vi "Estiban Shooter Code.vi"(9 "Cannon Height in Inches":dbl, 10 "Target Height in Inches":dbl, 11 "Distance to Shoot In Feet":dbl) -> (3 "Wheel RPM":dbl)   [LabVIEW 2011]
panel:
  out "Wheel RPS":dbl
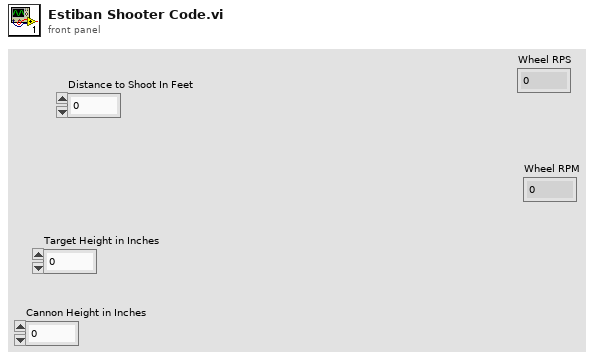
[diagram p1: front panel]
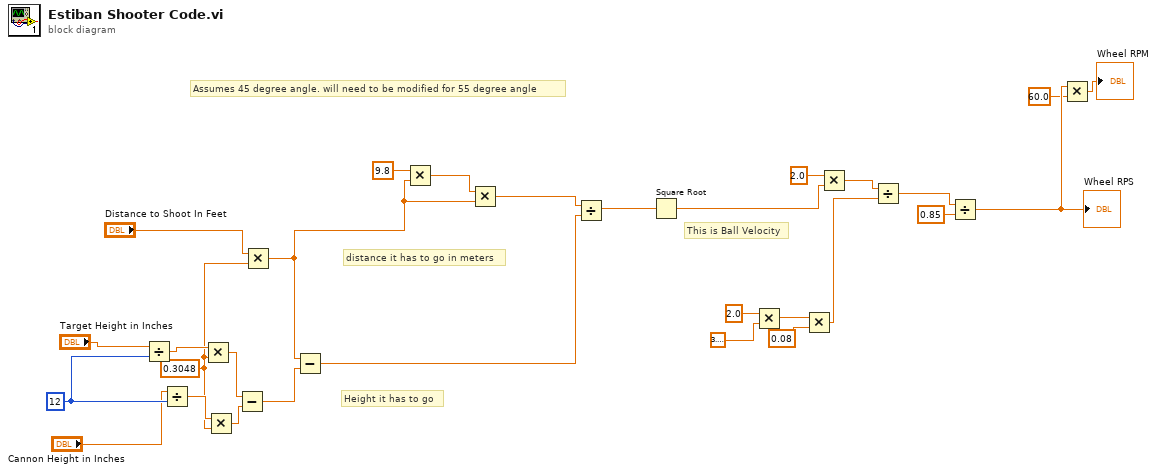
[diagram p0: block diagram]
diagram:
  w14 = 0.3048 ("y")
  w27 = 12
  # "distance it has to go in meters"
  # "Height it has to go"
  # "Assumes 45 degree angle. will need to be modified for 55 degree angle"
  # "This is Ball Velocity"
  n1 = Divide(x="Target Height in Inches", y=w27) -> (x/y=w25:dbl)
  n2 = Divide(x="Cannon Height in Inches", y=w27) -> (x/y=w22:dbl)
  n3 = Multiply(x=w25, y=w14) -> (x*y=w24:dbl)
  n4 = Multiply(x=w22, y=w14) -> (x*y=w23:dbl)
  n5 = Subtract(x=w24, y=w23) -> (x-y=w29:dbl)
  n6 = Multiply(x="Distance to Shoot In Feet", y=w14) -> (x*y=w15:dbl)
  n7 = Subtract(x=w15, y=w29) -> (x-y=w18:dbl)
  n8 = Multiply(x=9.8, y=w15) -> (x*y=w20:dbl)
  n9 = Multiply(x=w20, y=w15) -> (x*y=w19:dbl)
  n10 = Divide(x=w19, y=w18) -> (x/y=w17:dbl)
  n11 = Square Root(x=w17) -> (sqrt(x)=w12:dbl)
  n12 = Multiply(x=2.0, y=3.141592653589793) -> (x*y=w8:dbl)
  n13 = Multiply(x=w8, y=0.08) -> (x*y=w6:dbl)
  n14 = Multiply(x=2.0, y=w12) -> (x*y=w11:dbl)
  n15 = Divide(x=w11, y=w6) -> (x/y=w5:dbl)
  n16 = Divide(x=w5, y=0.85) -> (x/y=w2:dbl)
  "Wheel RPS" <- w2
  n17 = Multiply(x=w2, y=60.0) -> (x*y=→"Wheel RPM":dbl)
